vi "DAQ_Host_OPC UA.vi"() -> ()   [LabVIEW 2017]
uses:
  <vilib>/OPCUA/controls/NodeId.ctl
  <vilib>/OPCUA/controls/Write Status.ctl
  <vilib>/Utility/file.llb/Read Delimited Spreadsheet (string).vi
  <vilib>/Utility/file.llb/Write Delimited Spreadsheet (string).vi
  <vilib>/OPCUA/client/Multiple Write Double Array.vi
  <vilib>/Utility/file.llb/Write Delimited Spreadsheet (DBL).vi
  <resource>/objmgr/ni.dex.rc
  <vilib>/OPCUA/NI OPC UA Client.lvlib
panel:
  in  "Node Status":u32
  in  "Time Stamp":timestamp
  in  "Error In":errorcluster
  out "Error Out":errorcluster
  in  "Stop DAQ":bool
  out "DAQ?":bool
  out "Available Elements for Reading":i32
  out "Number of Disconnections":u32
  out "System Loop Time (ms)":u32
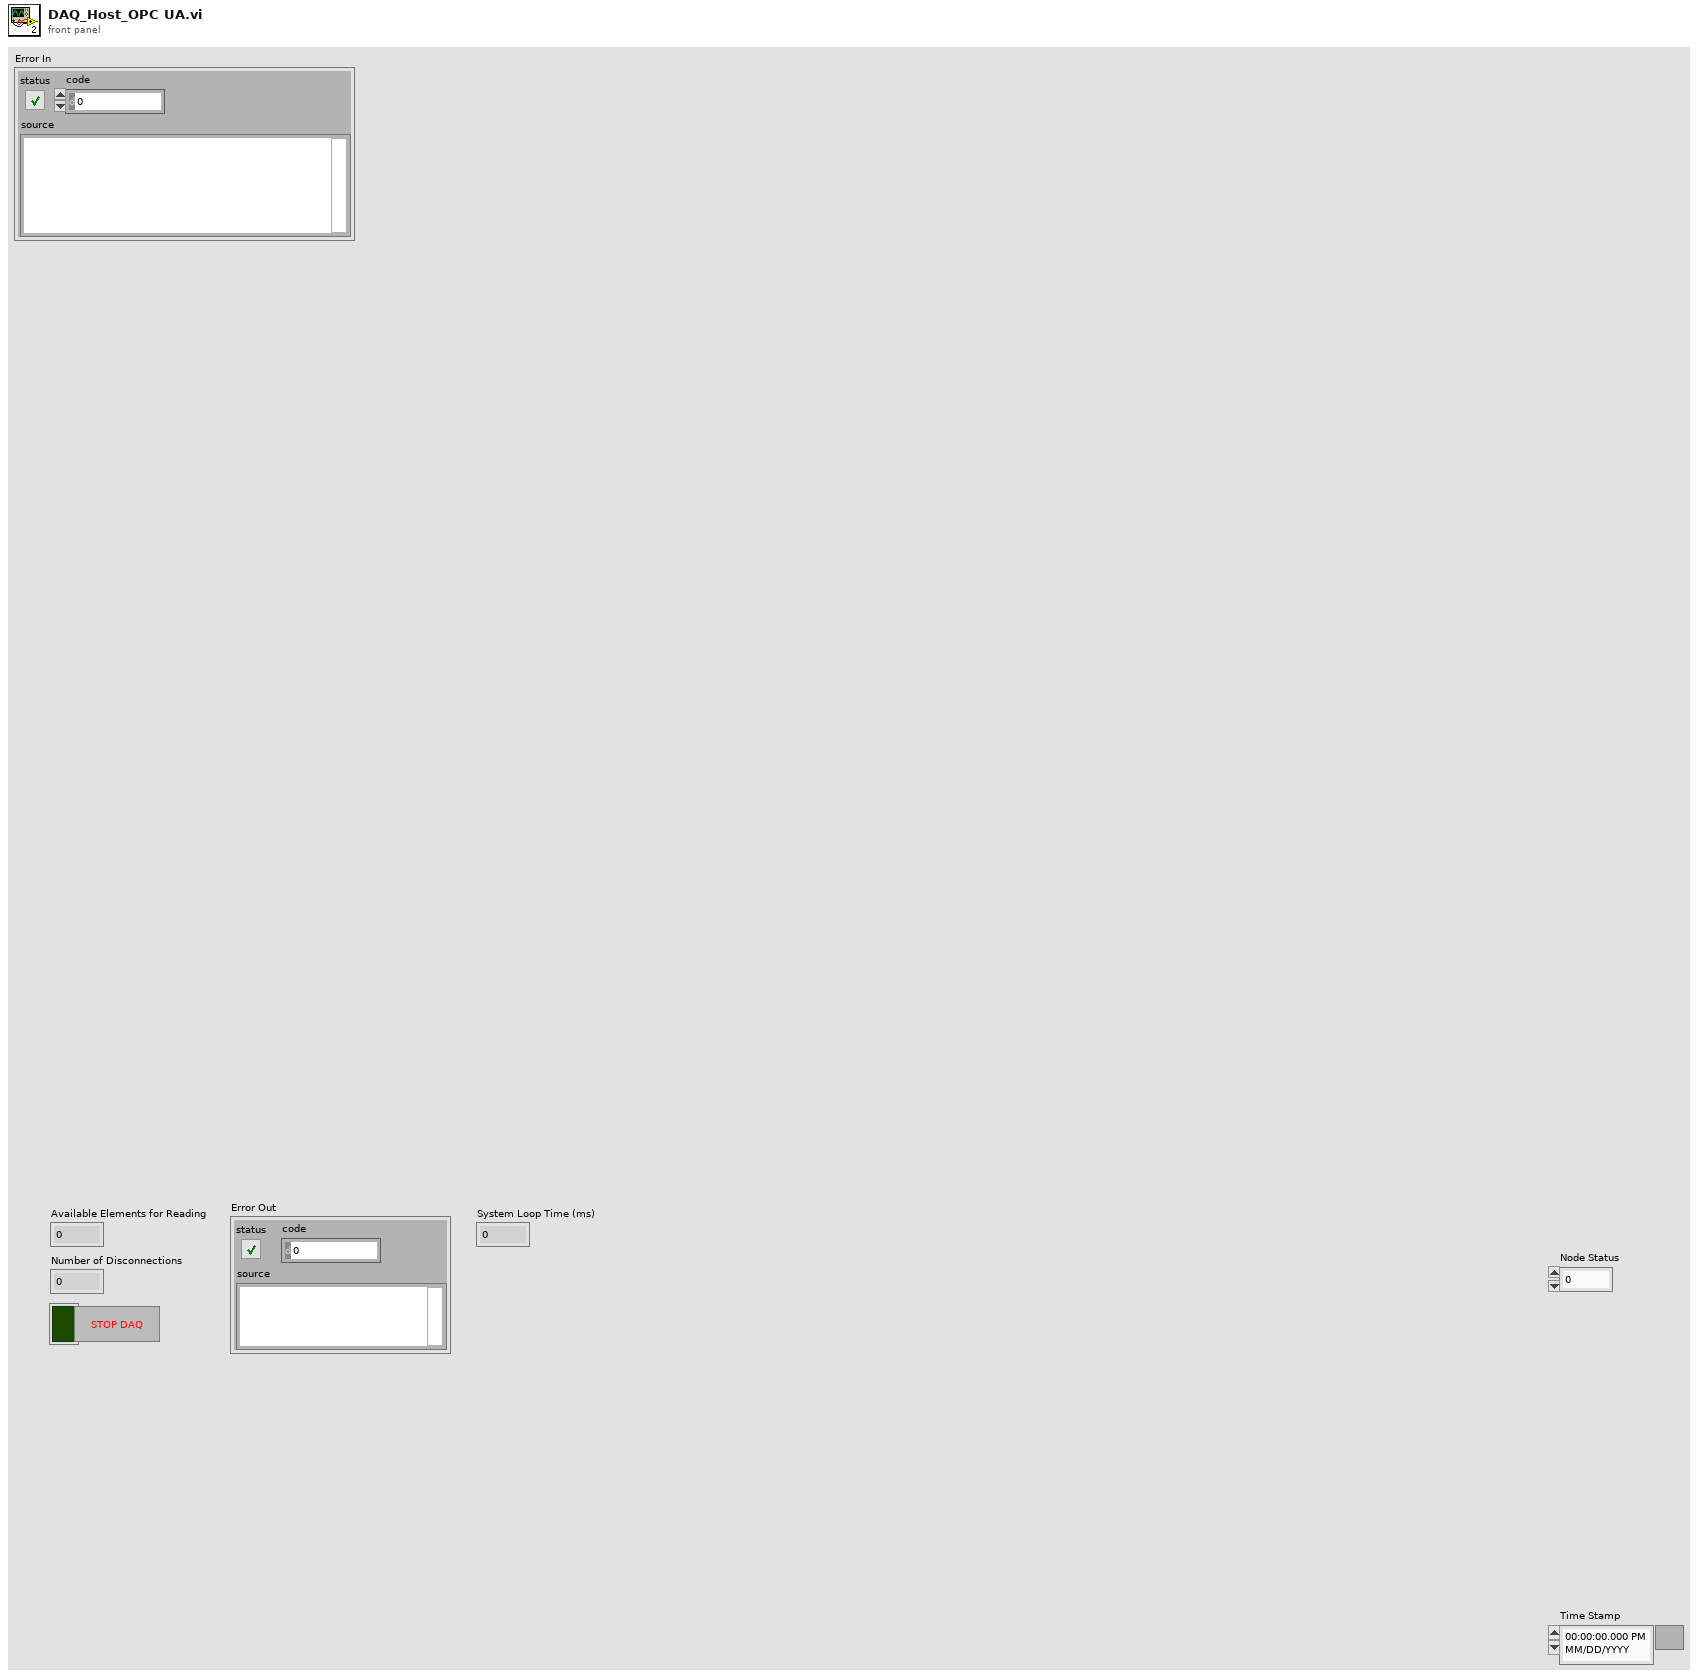
[diagram p1: front panel]
types:
  T1 = typedef "OPC UA Client Refnum.ctl" = refnum<k21>
  T2 = typedef "NodeId.ctl" = string
  T3 = typedef "Write Status.ctl" = u32
  T4 = cluster{"node ID":T2, "value":dbl[], "timestamp (current time)":timestamp, "node status":T3}
  T5 = cluster{"node ID":T2, "value":dbl[], "timestamp (current time)":timestamp, "node status":T3}[]
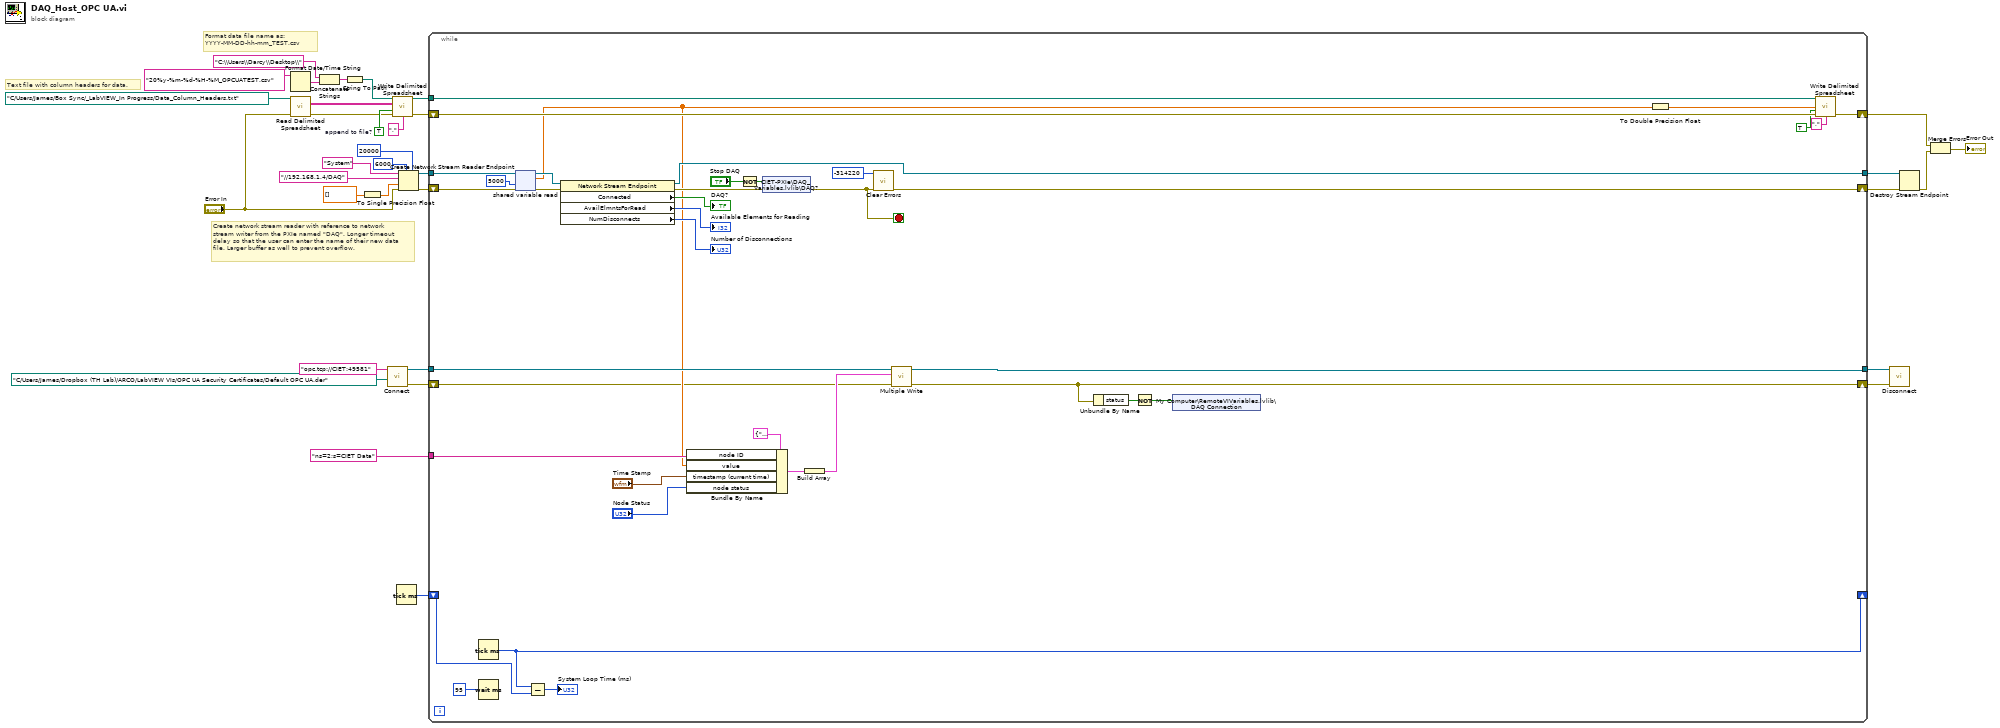
[diagram p0: block diagram]
diagram:
  w21 = TRUE  # append to file?
  # "Format data file name as:\nYYYY-MM-DD-hh-mm_TEST.csv"
  # "Create network stream reader with reference to network\nstream writer from the PXIe named \"DAQ\". Longer timeout\ndelay so that the user can enter the name of their new data\nfile. Larger buffer as well to prevent overflow."
  # "Text file with column headers for data."
  n1 = Format Date/Time String(time format string (%c)="20%y-%m-%d-%H-%M_OPCUATEST.csv") -> (date/time string=w11:string)  [unwired: 2 in]
  n2 = call-poly <vilib>:"Read Delimited Spreadsheet.vi"("file path (dialog if empty)"=path "C:/Users/James/Box Sync/_LabVIEW_In Progress/Data_Column_Headers.txt", "error in (no error)"="Error In") -> ("all rows"=w24:string[][], "error out"=w19:errorcluster)  [unwired: 8 in, 4 out]
  n3 = Concatenate Strings("C:\\Users\\Darcy\\Desktop\\" ("string"), w11) -> (w13:string)
  n4 = String To Path(string=w13) -> (path=w10:path)
  n5 = To Single Precision Float(number=dbl[] []) -> (single precision float=w32:sgl[])
  n6 = call <vilib>:"Connect.vi"("client certificate file"=path "C:/Users/James/Dropbox (TH Lab)/ARCO/LabVIEW VIs/OPC UA Security Certificates/Default OPC UA.der", "server endpoint URL"="opc.tcp://CIET:49581") -> ("error out"=w4:errorcluster, "OPC UA client refnum out"=w5:T1)  [unwired: 7 in, 1 out]
  n7 = call-poly <vilib>:"Write Delimited Spreadsheet.vi"("file path (dialog if empty)"=w10, "2D data"=w24, "append to file? (new file:F)"=w21, "error in (no error)"=w19, "delimiter (\\t)"=",") -> ("new file path (Not A Path if cancelled)"=w20:path, "error out"=w18:errorcluster)  [unwired: 9 in]
  n8 = Tick Count (ms)() -> (millisecond timer value=w8:u32)
  n9 = Create Network Stream Reader Endpoint(5:20000 ("timeout in ms (-1)"), 7:6000 ("reader buffer size"), 8:"Error In", 9:w32, 10:"//192.168.1.4/DAQ" ("writer url"), 11:"System" ("reader name")) -> (0:w29:errorcluster, 3:w28:refnum<k21>)  [unwired: 1 in]
  n10 = while {
    shift-right: [w61] -> w27
    shift-left: w29 -> [w69]
    tunnel: w28 -> [w70]
    tunnel: [w60] -> w26
    tunnel: w20 -> [w57]
    shift-right: [w55] -> w17
    shift-left: w18 -> [w56]
    shift-right: [w50] -> _
    shift-left: w8 -> [w51]
    tunnel: w5 -> [w45]
    tunnel: "ns=2;s=CIET Data" -> [w44]
    tunnel: [w36] -> w2
    shift-right: [w35] -> w1
    shift-left: w4 -> [w42]
    stop <- w41 stop-if-true
    n11 = Tick Count (ms)() -> (millisecond timer value=w50:u32)
    n12 = Wait (ms)(milliseconds to wait=u32 95) -> ()  [unwired: 1 out]
    n13 = shared-variable-read(w70, w69, 5000 ("timeout ms (-1)")) -> (w66:refnum<k21>, w64:errorcluster, w43:sgl[])  [unwired: 1 out]
    n14 = Subtract(x=w50, y=w51) -> (x-y=→"System Loop Time (ms)":u32)
    n15 = property class="Network Stream Endpoint"(reference=w66, error in=w64) -> (reference out=w60:refnum<k21>, error out=w65:errorcluster, "Connected"=→"DAQ?":bool, "AvailElmntsForRead"=→"Available Elements for Reading":i32, "NumDisconnects"=→"Number of Disconnections":u32)
    n16 = Bundle By Name(cluster=T4 {"node ID"="", "value"=[], "timestamp (current time)"=timestamp(0 s since 1904-01-01), "node status"=0} ("request"), "node ID"=w44, "value"=w43, "timestamp (current time)"="Time Stamp", "node status"="Node Status") -> (w47:T4)
    n17 = Not(x="Stop DAQ") -> (.not. x?=w68:bool)
    n18 = shared-variable "CIET-PXIe\\DAQ_Variables.lvlib\\DAQ?"(w68, error in=w65) -> (error out=w41:errorcluster)
    n19 = Build Array(w47) -> (w46:T5)
    n20 = call <vilib>:"Clear Errors.vi"("error in (no error)"=w41, "specific error code to clear (0: all)"=-314220) -> ("error out"=w61:errorcluster)  [unwired: 4 in, 1 out]
    n21 = call-poly <vilib>:"Multiple Write.vi"("error in (no error)"=w42, "requests"=w46, "OPC UA client refnum in"=w45) -> ("error out"=w35:errorcluster, "OPC UA client refnum out"=w36:T1)  [unwired: 5 in, 2 out]
    n22 = Unbundle By Name(w35) -> ("status"=w40:bool)
    n23 = Not(x=w40) -> (.not. x?=w39:bool)
    n24 = shared-variable "My Computer\\RemoteVIVariables.lvlib\\DAQ Connection"(w39) -> ()  [unwired: 1 in, 1 out]
    n25 = To Double Precision Float(number=w43) -> (double precision float=w52:dbl[])
    n26 = call-poly <vilib>:"Write Delimited Spreadsheet.vi"("file path (dialog if empty)"=w57, "1D data"=w52, "append to file? (new file:F)"=TRUE, "error in (no error)"=w56, "delimiter (\\t)"="," ("delimiter (\\t)")) -> ("error out"=w55:errorcluster)  [unwired: 9 in, 1 out]
  }
  n27 = call <vilib>:"Disconnect.vi"("error in (no error)"=w1, "OPC UA client refnum in"=w2) -> ()  [unwired: 9 in, 1 out]
  n28 = Destroy Stream Endpoint(8:w27, 11:w26) -> (0:w16:errorcluster)
  n29 = Merge Errors(w17, w16) -> (→"Error Out":errorcluster)
